vi "Write and Read Multiple Registers Response.vi"(8 "error in":errorcluster, 10 "modbus data unit in":refnum<class "Modbus Data Unit.lvclass">) -> (0 "error out":errorcluster, 1 "Registers":u16[](array[numeric]), 2 "Byte Count":u8)   [LabVIEW 2021, in "Master Function Definition.lvclass"]
doc: "Decodes the response generated by the write and read multiple holding registers function."
uses:
  Master Function Definition.lvclass
  Modbus Data Unit/Modbus Data Unit.lvclass
  Modbus Data Unit/Modbus Data Unit.lvclass/Modbus Data Unit.ctl
  Master Function Definition.lvclass/Master Function Definition.ctl
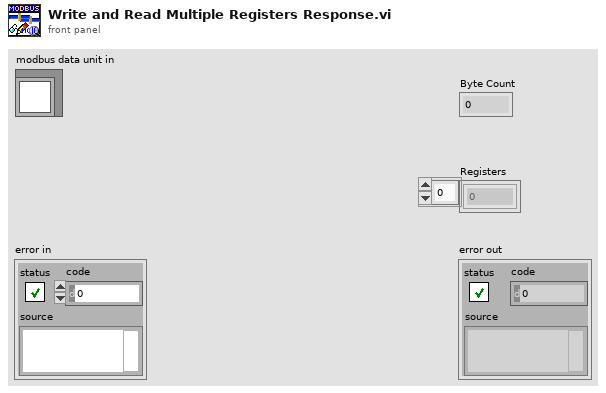
[diagram p1: front panel]
types:
  T1 = typedef "Modbus Data Unit.lvclass/Function.ctl" = u8
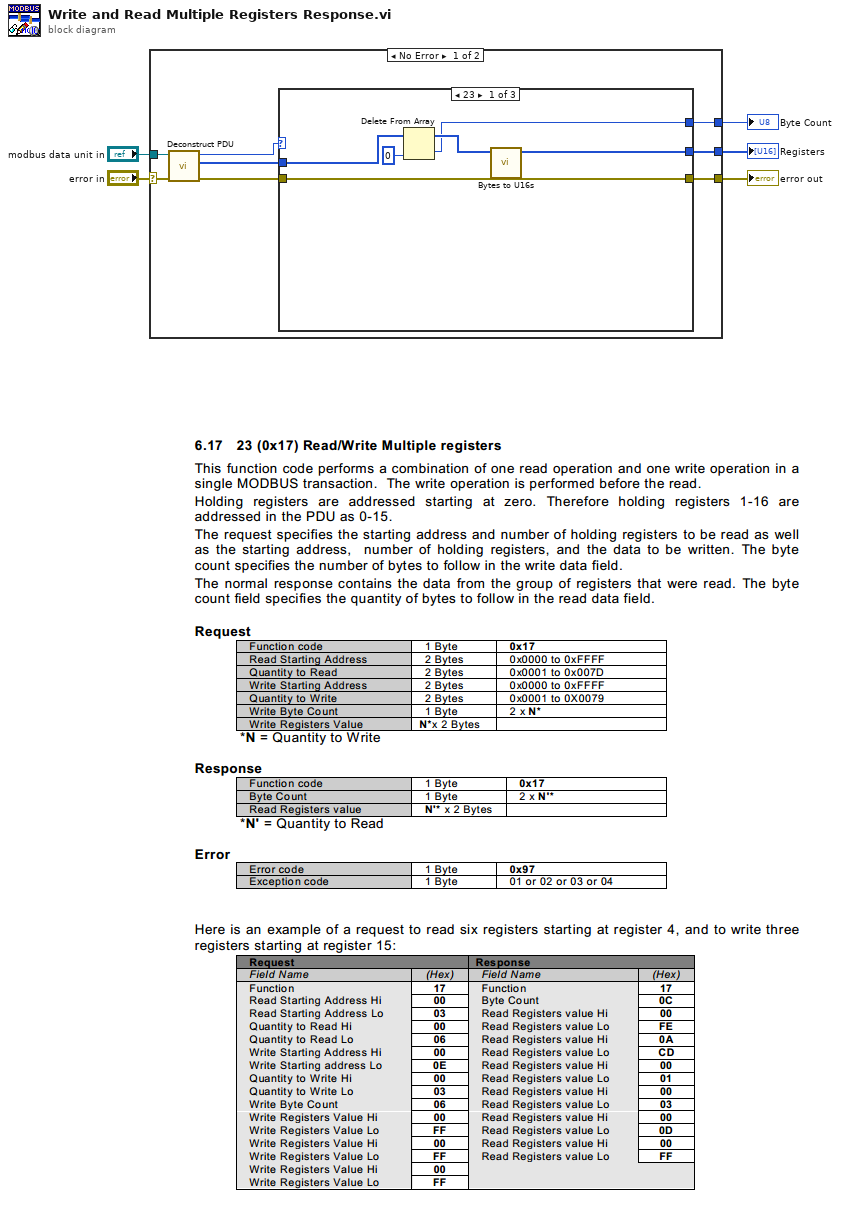
[diagram p0: block diagram]
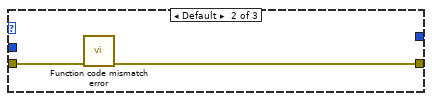
[diagram p2: hidden frame]
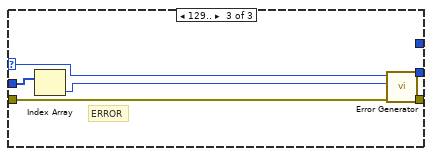
[diagram p3: hidden frame]
diagram:
  n1 = case shown="No Error" "error in" {
    selector: "error in" -> [w12 w27]
    tunnel: [w13 w27] -> w4
    tunnel: "modbus data unit in" -> [w10 _]
    tunnel: [w7 _] -> w2
    tunnel: [w6 _] -> w1
    frame No Error {
      n2 = call "Deconstruct PDU.vi"("error in"=w12, "modbus data unit in"=w10) -> ("error out"=w9:errorcluster, "data"=w11:u8[], "Function"=w8:T1)  [unwired: 7 in]
      n3 = case shown="23" w8 {
        selector: w8 -> [_ _ w22]
        tunnel: w9 -> [w19 w21 w23]
        tunnel: w11 -> [w16 _ w26]
        tunnel: [w19 w20 w25] -> w13
        tunnel: [w15 _ _] -> w7
        tunnel: [w14 _ _] -> w6
        frame 23 {
          n4 = Delete From Array(array=w16, index=0) -> (deleted portion=w15:u8, array with subset deleted=w17:u8[])  [unwired: 1 in]
          n5 = call "Bytes to U16s.vi"("Bytes"=w17) -> ("Registers"=w14:u16[])  [unwired: 10 in]
        }
        frame Default {
          n6 = call "Function code mismatch error.vi"("error in (no error)"=w21) -> ("error out"=w20:errorcluster)  [unwired: 10 in]
        }
        frame 129.. {
          # "ERROR"
          n7 = Index Array(array=w26) -> (element=w24:u8)  [unwired: 1 in]
          n8 = call "Error Generator.vi"("error in"=w23, "data return (error code)"=w24, "function return"=w22) -> ("error out"=w25:errorcluster)  [unwired: 8 in]
        }
      }
    }
    frame Error {
    }
  }
  "error out" <- w4
  "Byte Count" <- w2
  "Registers" <- w1
